vi "test.vi"() -> ()   [LabVIEW 2017, in "ModBUS.lvlib" / "RTU.lvclass"]
uses:
  RTU.lvclass
panel:
  out "Finished 3":bool
  out "OK? 3":bool
  out "Data 3":i16[](array[numeric])
  in  "Data in: 3":u8[](array[numeric])=[1, 0, 25, 0, 3, 97, 0] format="%.0x"
  out "Data 2":i16[](array[numeric]) format="%.0x"
  out "Finished 2":bool
  out "OK? 2":bool
  in  "Data in: 2":u8[](array[numeric])=[1, 0, 25, 0, 3, 97, 0] format="%.0x"
  in  "Data in:":u8[](array[numeric])=[1, 0, 25, 0, 3, 97, 0] format="%.0x"
  out "Data":i16[](array[numeric])
  out "OK?":bool
  out "Finished":bool
  # "11 03 06 AE41 5652 4340 49AD"
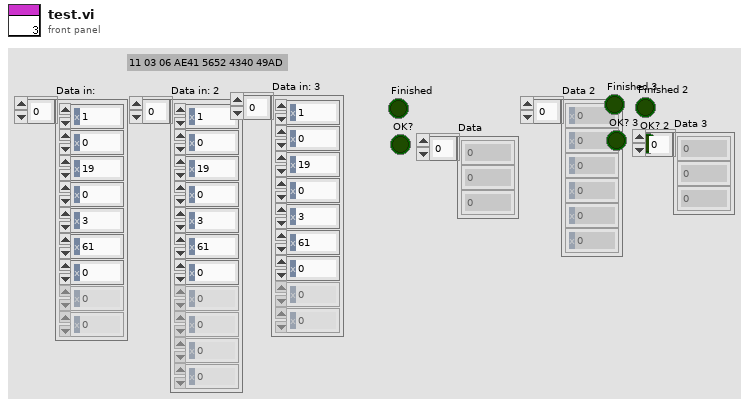
[diagram p1: front panel]
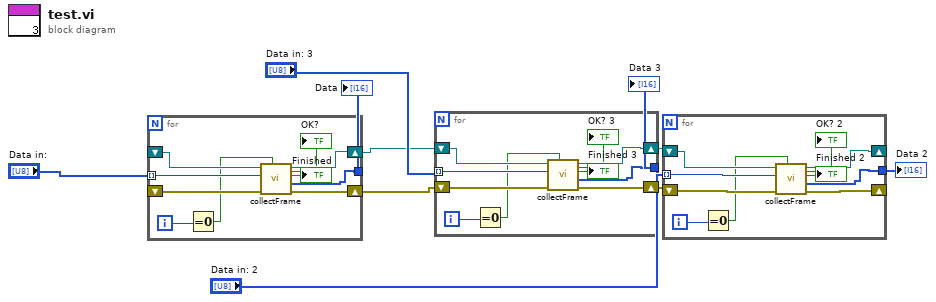
[diagram p0: block diagram]
diagram:
  n1 = for {
    shift-right: [w20] -> w1
    shift-left: _ -> [w19]
    tunnel: [w18] -> w9
    shift-right: [w17] -> w2
    shift-left: _ -> [w16]
    tunnel: "Data in:" -> [w13] mode=indexing
    i -> [w12]
    n2 = Equal To 0?(x=w12) -> (x = 0?=w11:bool)
    n3 = call-dynamic "collectFrame.vi"("Reset"=w11, "error in (no error)"=w19, "byte"=w13, "RTU in"=w16) -> ("error out"=w20:errorcluster, "Data"=w18:i16[], "Finished"=→"Finished":bool, "RTU out"=w17:refnum<class "RTU.lvclass">, "OK?"=→"OK?":bool)  [unwired: 3 in]
  }
  "Data" <- w9
  n4 = for {
    shift-right: [w30] -> w4
    shift-left: w1 -> [w29]
    tunnel: [w28] -> w6
    shift-right: [w27] -> w3
    shift-left: w2 -> [w26]
    tunnel: "Data in: 3" -> [w23] mode=indexing
    i -> [w22]
    n5 = Equal To 0?(x=w22) -> (x = 0?=w21:bool)
    n6 = call-dynamic "collectFrame.vi"("Reset"=w21, "error in (no error)"=w29, "byte"=w23, "RTU in"=w26) -> ("error out"=w30:errorcluster, "Data"=w28:i16[], "Finished"=→"Finished 3":bool, "RTU out"=w27:refnum<class "RTU.lvclass">, "OK?"=→"OK? 3":bool)  [unwired: 3 in]
  }
  "Data 3" <- w6
  n7 = for {
    shift-right: [w40] -> _
    shift-left: w4 -> [w39]
    tunnel: [w38] -> w7
    shift-right: [w37] -> _
    shift-left: w3 -> [w36]
    tunnel: "Data in: 2" -> [w33] mode=indexing
    i -> [w32]
    n8 = Equal To 0?(x=w32) -> (x = 0?=w31:bool)
    n9 = call-dynamic "collectFrame.vi"("Reset"=w31, "error in (no error)"=w39, "byte"=w33, "RTU in"=w36) -> ("error out"=w40:errorcluster, "Data"=w38:i16[], "Finished"=→"Finished 2":bool, "RTU out"=w37:refnum<class "RTU.lvclass">, "OK?"=→"OK? 2":bool)  [unwired: 3 in]
  }
  "Data 2" <- w7
